vi "Pcre2PatternInfoNameTable.vi"(8 "error in":errorcluster, 11 "pCode":u64 format="%.0x") -> (0 "error out":errorcluster, 1 "Numbers":i32[](array[numeric]), 2 "Names":string[](array[string]), 3 "pCode":u64 format="%.0x")   [LabVIEW 2021, in "libpcre2-8.lvlib"]
uses:
  libpcre2-8.lvlib
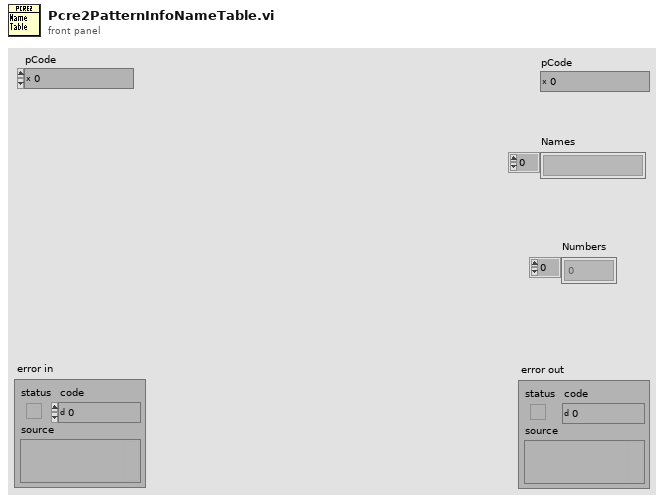
[diagram p1: front panel]
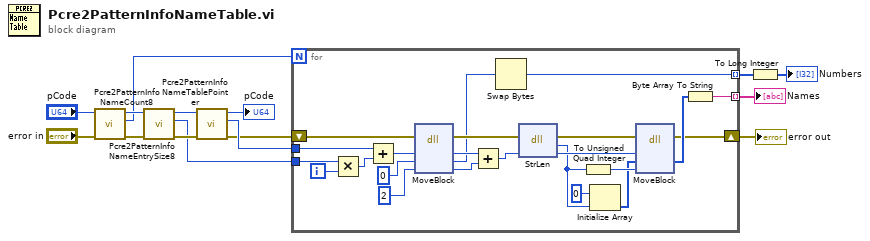
[diagram p0: block diagram]
diagram:
  n1 = call "Pcre2PatternInfoNameCount8.vi"("error in"="error in", "pCode"="pCode") -> ("error out"=w11:errorcluster, "NameCount"=w1:i32, "pCode"=w15:u64)  [unwired: 7 in]
  n2 = call "Pcre2PatternInfoNameEntrySize8.vi"("error in"=w11, "pCode"=w15) -> ("error out"=w10:errorcluster, "NameEntrySize"=w8:u64, "pCode"=w14:u64)  [unwired: 7 in]
  n3 = call "Pcre2PatternInfoNameTablePointer.vi"("error in"=w10, "pCode"=w14) -> ("error out"=w6:errorcluster, "pNameTable"=w7:u64, "pCode"=→"pCode":u64)  [unwired: 7 in]
  n4 = for {
    N: w1 -> [_]
    tunnel: w8 -> [w37]
    tunnel: w7 -> [w36]
    tunnel: [w16] -> w5 mode=indexing
    tunnel: [w24] -> w2 mode=indexing
    shift-right: [w23] -> w3
    shift-left: w6 -> [w25]
    i -> [w18]
    n5 = Multiply(x=w37, y=w18) -> (x*y=w22:u64)
    n6 = Add(x=w36, y=w22) -> (x+y=w35:u64)
    n7 = dll-call lib="LabVIEW" fn="MoveBlock"(error in=w25, "pointerSrc"=w35, "pointerDest"=i16 0 ("size"), "size"=u64 2) -> (error out=w27:errorcluster, "pointerSrc"=w33:u64, "pointerDest"=w17:i16, "size"=w32:u64)  [unwired: 3 in, 1 out]
    n8 = Add(x=w33, y=w32) -> (x+y=w26:u64)
    n9 = Swap Bytes(anything=w17) -> (byte swapped=w16:i16)
    n10 = dll-call lib="LabVIEW" fn="StrLen"(error in=w27, "s"=w26) -> (error out=w30:errorcluster, "size"=w20:i32, "s"=w31:u64)  [unwired: 2 in, 1 out]
    n11 = To Unsigned Quad Integer(1:w20) -> (0:w28:u64)
    n12 = Initialize Array(u8 0 ("U8"), w20) -> (w19:u8[])
    n13 = dll-call lib="LabVIEW" fn="MoveBlock"(error in=w30, "pointerSrc"=w31, "pointerDest"=w19, "size"=w28) -> (error out=w23:errorcluster, "pointerDest"=w29:u8[])  [unwired: 5 in, 1 out]
    n14 = Byte Array To String(unsigned byte array=w29) -> (string=w24:string)
  }
  "error out" <- w3
  "Names" <- w2
  n15 = To Long Integer(number=w5) -> (32bit integer=→"Numbers":i32[])
